vi "Finish.vi"   [LabVIEW 2015]
doc: "This VI is called just before exiting. It is expected to close I/O refnum, save collected data, etc."
uses:
  <vilib>/Rock Robotics/WPI/Utilities/WPI_GetSetVariantRefNum.vi
types:
  T1 = typedef "WPI_MotorControlDeviceRef.ctl" = cluster{"DeviceStatus":errorcluster, "Type":T2, "PWM":cluster{"PWM Channel":T3, "DeadBand":T4}, "CAN":cluster{"Device Number":u8, "Control Mode":T5, "Semaphore":T6, "Max Vout":dbl, "TalonSRX Control Mode":T7}, "Invert":bool}
  T2 = typedef "WPI_MotorControlType.ctl" = enum16{"PWM", "CAN", "CANTalonSRX"}
  T3 = typedef "FPGA_DIOPWMChannel.ctl" = enum8{"PWM 0", "PWM 1", "PWM 2", "PWM 3", "PWM 4", "PWM 5", "PWM 6", "PWM 7", "PWM 8", "PWM 9", "PWM MXP 0", "PWM MXP 1", "PWM MXP 2", "PWM MXP 3", "PWM MXP 4", "PWM MXP 5", "PWM MXP 6", "PWM MXP 7", "PWM MXP 8", "PWM MXP 9", "Invalid"}
  T4 = typedef "WPI_PWMDeadband.ctl" = cluster{"Name":string, "maxPositivePwm":i32, "minPositivePwm":i32, "centerPwm":i32, "maxNegativePwm":i32, "minNegativePwm":i32, "angularRange":u16}
  T5 = typedef "WPI_CANJaguar_ControlMode.ctl" = enum8{"Percent VBus", "Current", "Speed", "Position", "Voltage"}
  T6 = typedef "Semaphore RefNum" = refnum<k1>
  T7 = typedef "WPI_CANTalonSRX_APIControlMode.ctl" = enum8{"Percent VBus", "Speed", "Position", "Slave", "Unchanged / Invalid", "Voltage Compensation", "Current", "Motion Profile"}
  T8 = typedef "WPI_JoystickDevRef.ctl" = cluster{"Device":T9}
  T9 = typedef "WPI_JoystickDeviceEnum.ctl" = enum16{"USB 0", "USB 1", "USB 2", "USB 3", "USB 4", "USB 5"}
  T10 = typedef "WPI_RobotDriveDevRef.ctl" = cluster{"DevStatus":errorcluster, "Motors[]":T1[], "Square Inputs":bool, "Max Output":dbl}
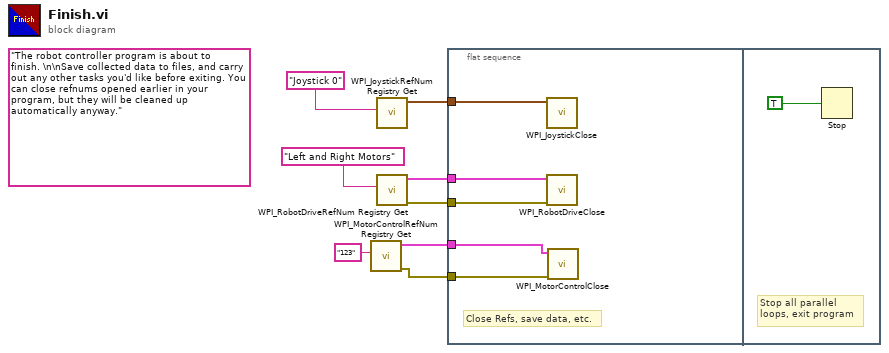
[diagram p0: block diagram]
diagram:
  (unwired) "The robot controller program is about to finish. \n\nSave collected data to files, and carry out any other tasks you'd like before exiting. You can close refnums opened earlier in your program, but they will be cleaned up automatically anyway."
  n1 = call <vilib>:"WPI_MotorControlRefNum Registry Get.vi"("refnum name"="123") -> ("error out"=w2:errorcluster, "MotorControlDevRef"=w3:T1)  [unwired: 9 in]
  n2 = call <vilib>:"WPI_JoystickRefNum Registry Get.vi"("refnum name"="Joystick 0") -> ("JoystickDevRef"=w5:T8)  [unwired: 1 in, 9 out]
  n3 = call <vilib>:"WPI_RobotDriveRefNum Registry Get.vi"("refnum name"="Left and Right Motors") -> ("error out"=w1:errorcluster, "RobotDriveDevRef"=w6:T10)  [unwired: 1 in, 8 out]
  n4 = flat-sequence {
    tunnel: w6 -> [w13]
    tunnel: w5 -> [w12]
    tunnel: w3 -> [w11]
    tunnel: w2 -> [w10]
    tunnel: w1 -> [w9]
    frame #0 {
      # "Close Refs, save data, etc."
      n5 = call <vilib>:"WPI_JoystickClose.vi"("JoystickDevRef"=w12) -> ()  [unwired: 11 out]
      n6 = call <vilib>:"WPI_RobotDriveClose.vi"("error in (no error)"=w9, "RobotDriveDevRef"=w13) -> ()  [unwired: 10 out]
      n7 = call <vilib>:"WPI_MotorControlClose.vi"("error in (no error)"=w10, "MotorControlDevRef"=w11) -> ()  [unwired: 9 in, 1 out]
    }
    frame #1 {
      # "Stop all parallel\nloops, exit program"
      n8 = Stop(stop? (T)=TRUE ("Quit")) -> ()
    }
  }
